vi "FGV-GlobalEventRef.vi"(6 "Operation":enum16{"Create", "Read", "Destroy"}(ring), 8 "error in (no error)":errorcluster, 9 "Timeout In ms (5000 ms)":i32=5000, 10 "Force Destroy?":bool) -> (0 "error out":errorcluster, 3 "Event":refnum<user-event>)   [LabVIEW 2017, in "Communicable State Machine.lvlib"]
doc: "### FGV-GlobalEventRef.vi\n\n-- <b>Controls</b> --\n- <b>Create(F)</b>:\n\n-- <b>Indicators</b> --\n- <b>CSM Global Log Event</b>:"
uses:
  Communicable State Machine.lvlib
  Typedef/_CSM_GlobalLog_MSG.ctl
  Typedef/_CSM_Response Source Message.ctl
  Typedef/_CSM_GlobalLog_MSG_TYPE.ctl
  ChangeFlag/ChangeFlag-Write.vi
  Utility/Random Change Flag.vi
  ChangeFlag/ChangeFlagDB.vi
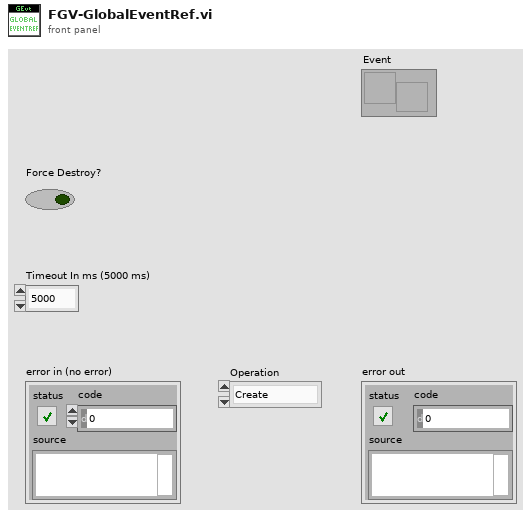
[diagram p1: front panel]
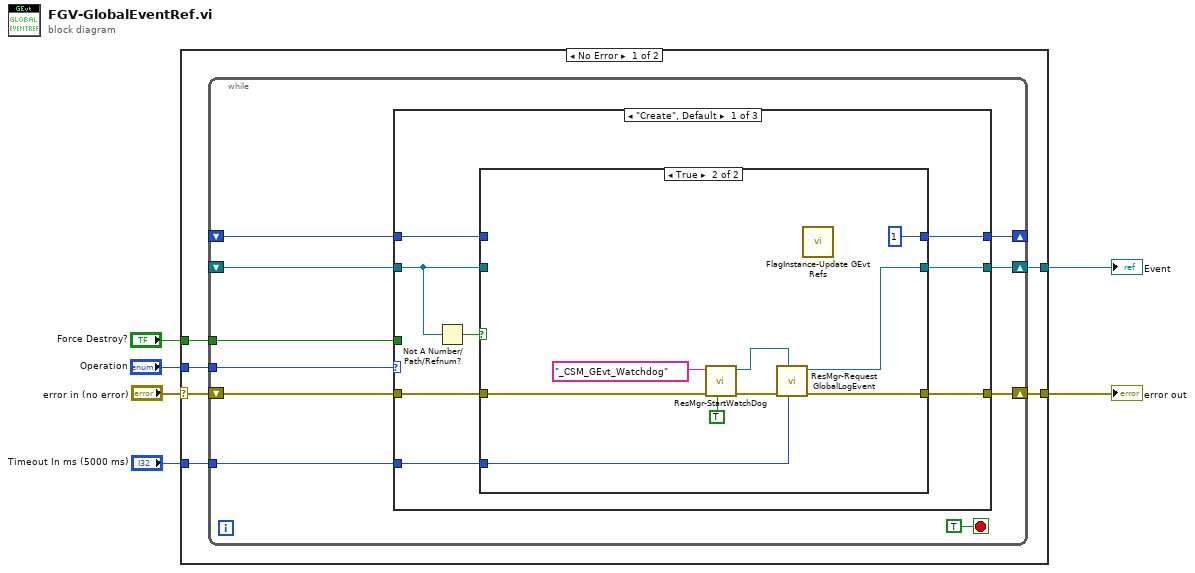
[diagram p0: block diagram]
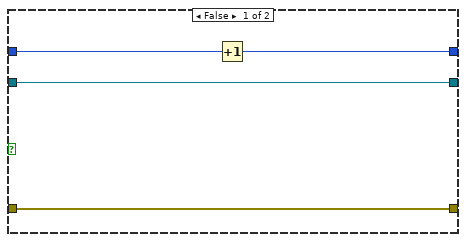
[diagram p2: hidden frame]
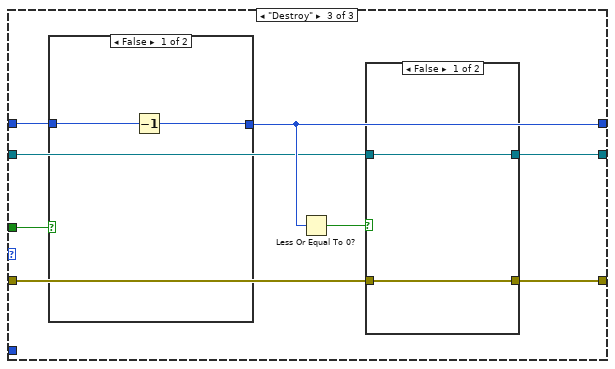
[diagram p4: hidden frame]
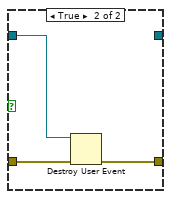
[diagram p5: hidden frame]
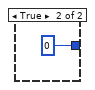
[diagram p6: hidden frame]
diagram:
  n1 = case shown="No Error" "error in (no error)" {
    selector: "error in (no error)" -> [w11 w63]
    tunnel: [w12 _] -> w6
    tunnel: [w10 w63] -> w4
    tunnel: "Operation" -> [w9 _]
    tunnel: "Timeout In ms (5000 ms)" -> [w8 _]
    tunnel: "Force Destroy?" -> [w7 _]
    frame No Error {
      n2 = while {
        shift-right: [w20] -> w10
        shift-left: w11 -> [w21]
        shift-right: [w22] -> w12
        shift-left: _ -> [w18]
        tunnel: w9 -> [w16]
        tunnel: w8 -> [w17]
        tunnel: w7 -> [w13]
        shift-right: [w15] -> _
        shift-left: _ -> [w14]
        stop <- TRUE stop-if-true
        n3 = case shown="\"Create\", Default" w16 {
          tunnel: [w28 w45 w47] -> w22
          tunnel: w21 -> [w30 w44 w51]
          tunnel: [w29 w44 w50] -> w20
          tunnel: w18 -> [w25 w45 w49]
          tunnel: w17 -> [w27 _ _]
          tunnel: [w24 w46 w52] -> w15
          tunnel: w14 -> [w23 w46 w53]
          tunnel: w13 -> [_ _ w54]
          frame "Create", Default {
            n4 = Not A Number/Path/Refnum?(number/path/refnum=w25) -> (NaN/Path/Refnum?=w26:bool)
            n5 = case shown="True" w26 {
              tunnel: w30 -> [w33 w40]
              tunnel: [w33 w39] -> w29
              tunnel: [w34 w38] -> w28
              tunnel: w27 -> [_ w37]
              tunnel: w25 -> [w34 _]
              tunnel: [w31 1] -> w24
              tunnel: w23 -> [w32 _]
              frame False {
                n6 = Increment(x=w32) -> (x+1=w31:i32)
              }
              frame True {
                n7 = call "ResMgr-StartWatchDog.vi"("Force?"=TRUE, "error in (no error)"=w40, "ModuleName"="_CSM_GEvt_Watchdog") -> ("error out"=w42:errorcluster, "WatchDogQ"=w41:refnum<queue>)  [unwired: 7 in]
                n8 = call "ResMgr-Request GlobalLogEvent.vi"("Timeout In ms (5000 ms)"=w37, "WatchDogQ"=w41, "Error In"=w42) -> ("error out"=w39:errorcluster, "GlobalLogEvent"=w38:refnum<user-event>)  [unwired: 7 in]
                n9 = call "FlagInstance-Update GEvt Refs.vi"() -> ()  [unwired: 10 in, 2 out]
              }
            }
          }
          frame "Read" {
          }
          frame "Destroy" {
            n10 = case shown="False" w54 {
              tunnel: [w60 0] -> w52
              tunnel: w53 -> [w61 _]
              frame False {
                n11 = Decrement(x=w61) -> (x-1=w60:i32)
              }
              frame True {
              }
            }
            n12 = Less Or Equal To 0?(x=w52) -> (x <= 0?=w48:bool)
            n13 = case shown="False" w48 {
              tunnel: w51 -> [w56 w59]
              tunnel: [w56 w58] -> w50
              tunnel: w49 -> [w55 w57]
              tunnel: [w55 _] -> w47
              frame False {
              }
              frame True {
                n14 = Destroy User Event(user event=w57, error in=w59) -> (error out=w58:errorcluster)
              }
            }
          }
        }
      }
    }
    frame Error {
    }
  }
  "Event" <- w6
  "error out" <- w4
